vi "LM model function and gradient (Gaussian (X) 1-Exp).vi"(3 "output control":T1, 4 "data":variant, 5 "X":dbl[](array[numeric]), 6 "a":dbl[](array[numeric])) -> (0 "error out":errorcluster, 1 "f'(X,a)":dbl[][](array[numeric]), 2 "f(X,a)":dbl[](array[numeric]))   [LabVIEW 2021, in "Fits.lvlib"]
doc: "This template is the starting point for creating a model function to be passed to the Nonlinear Curve Fit.vi."
uses:
  <vilib>/gmath/NumericalOptimization/LM_output select.ctl
  Fits.lvlib
  <vilib>/gmath/NI_Gmath.lvlib
  <vilib>/gmath/NI_AAL_MathFunc.lvlib
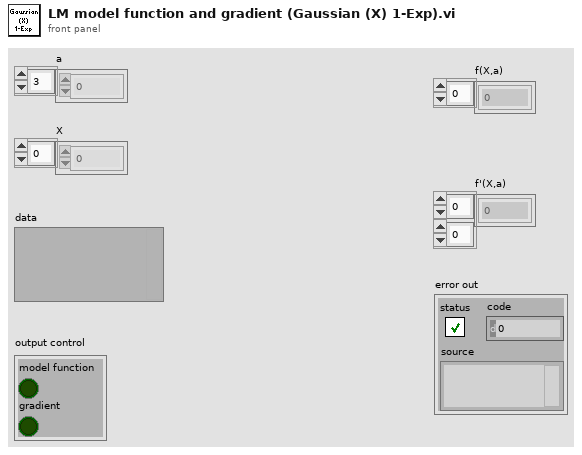
[diagram p1: front panel]
types:
  T1 = typedef "NI_Gmath.lvlib/LM_output select.ctl" = cluster{"model function":bool, "gradient":bool}
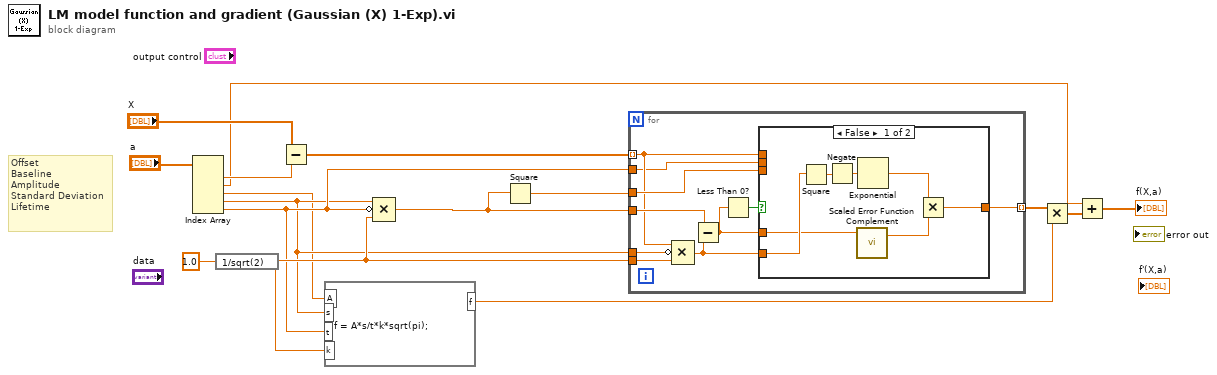
[diagram p0: block diagram]
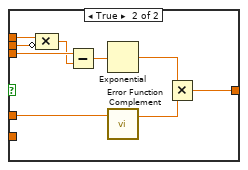
[diagram p2: hidden frame]
diagram:
  # "Offset\nBaseline\nAmplitude\nStandard Deviation\nLifetime"
  n1 = Index Array(array="a") -> (element #1=w13:dbl, element #2=w1:dbl, element #3=w3:dbl, element #4=w4:dbl, element #5=w5:dbl)  [unwired: 5 in]
  n2 = expression code="1/sqrt(2)"(1.0) -> (w9:dbl)
  n3 = Subtract(x="X", y=w13) -> (x-y=w14:dbl[])
  n4 = formula code="f = A*s/t*k*sqrt(pi);"("k"=w9, "A"=w3, "s"=w4, "t"=w5) -> ("f"=w7:dbl)
  n5 = Compound Arithmetic op=MULTIPLY(w4, invert w5, w9) -> (w11:dbl)
  n6 = Square(x=w11) -> (x^2=w10:dbl)
  n7 = for {
    tunnel: w14 -> [w21] mode=indexing
    tunnel: w5 -> [w20]
    tunnel: w11 -> [w23]
    tunnel: w10 -> [w25]
    tunnel: w9 -> [w22]
    tunnel: [w24] -> w8 mode=indexing
    tunnel: w4 -> [w19]
    n8 = Compound Arithmetic op=MULTIPLY(w21, invert w19, w22) -> (w18:dbl)
    n9 = Subtract(x=w23, y=w18) -> (x-y=w17:dbl)
    n10 = Less Than 0?(x=w17) -> (x < 0?=w26:bool)
    n11 = case shown="False" w26 {
      tunnel: w25 -> [_ w42]
      tunnel: w21 -> [_ w36]
      tunnel: [w30 w38] -> w24
      tunnel: w17 -> [w28 w37]
      tunnel: w20 -> [_ w34]
      tunnel: w18 -> [w29 _]
      frame False {
        n12 = Square(x=w29) -> (x^2=w33:dbl)
        n13 = Negate(x=w33) -> (-x=w27:dbl)
        n14 = call <vilib>:"Scaled Error Function Complement.vi"("x"=w28) -> ("scaled erfc(x)"=w31:dbl)  [unwired: 2 in]
        n15 = Exponential(1:w27) -> (0:w32:dbl)
        n16 = Multiply(x=w32, y=w31) -> (x*y=w30:dbl)
      }
      frame True {
        n17 = Compound Arithmetic op=MULTIPLY(w36, invert w34) -> (w35:dbl)
        n18 = Subtract(x=w42, y=w35) -> (x-y=w41:dbl)
        n19 = Exponential(1:w41) -> (0:w40:dbl)
        n20 = call <vilib>:"Error Function Complement.vi"("x"=w37) -> ("1 - erf(x)"=w39:dbl)  [unwired: 2 in]
        n21 = Multiply(x=w40, y=w39) -> (x*y=w38:dbl)
      }
    }
  }
  n22 = Multiply(x=w8, y=w7) -> (x*y=w6:dbl[])
  n23 = Add(x=w1, y=w6) -> (x+y=→"f(X,a)":dbl[])
